vi "Create.vi"() -> (8 "Tosca":refnum<class "Parameters.lvclass">)   [LabVIEW 2020, in "Parameters.lvclass"]
uses:
  Parameters.lvclass
  Parameters.lvclass/Parameters.ctl
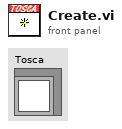
[diagram p1: front panel]
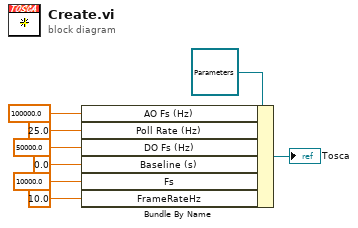
[diagram p0: block diagram]
diagram:
  n1 = Bundle By Name(cluster=refnum<class "Parameters.lvclass"> refnum ("Tosca"), "AO Fs (Hz)"=100000.0 ("Serialized.DAQ.AO Fs (Hz)"), "Poll Rate (Hz)"=25.0 ("Serialized.DAQ.Poll Rate (Hz)"), "DO Fs (Hz)"=50000.0 ("Serialized.DAQ.DO Fs (Hz)"), "Baseline (s)"=0.0 ("Serialized.DAQ.Baseline (s)"), "Fs"=10000.0 ("Serialized.AI.Fs"), "FrameRateHz"=10.0 ("Serialized.Imaging.FrameRateHz")) -> (→"Tosca":refnum<class "Parameters.lvclass">)
